vi "IniDataRd TDC.vi"(8 "error in":errorcluster, 10 "MODBUS section":string="Modbus", 11 "INI file path":path=path "C:/Users/User/Desktop/YDX701_TDC/iniData/TDC_IniData.ini") -> (0 "error out":errorcluster, 2 "MODBUS Para":T1={"COMPort"="COM4", "Slave Address"=1, " Baud"=9600, "Timeout"=100})   [LabVIEW 2019]
uses:
  <vilib>/Utility/config.llb/Read Key (U32).vi
  <vilib>/Utility/config.llb/Read Key (String).vi
  <vilib>/Utility/config.llb/NI_LVConfig.lvlib
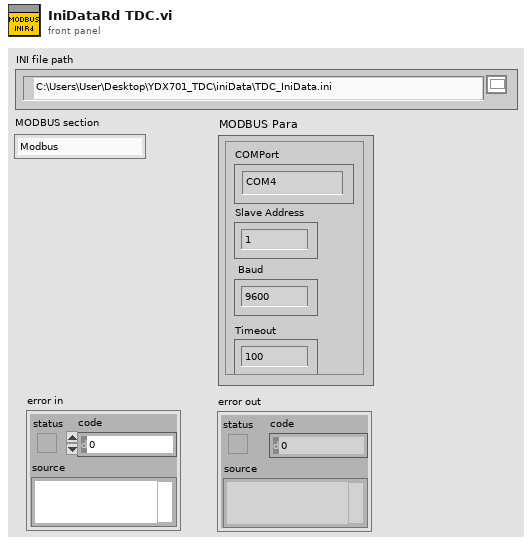
[diagram p1: front panel]
types:
  T1 = cluster{"COMPort":string, "Slave Address":u32, " Baud":u32, "Timeout":u32}
  T2 = typedef "NI_LVConfig.lvlib/Config Data RefNum.ctl" = refnum<k1>
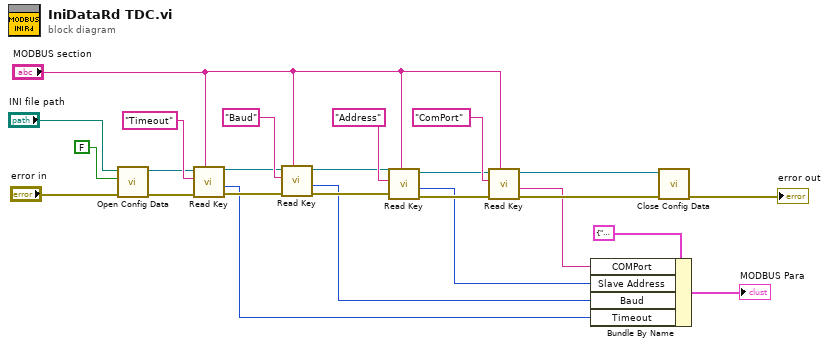
[diagram p0: block diagram]
diagram:
  n1 = call <vilib>:"Open Config Data.vi"("error in (no error)"="error in", "create file if necessary (T)"=FALSE ("create file if necessary? (T)"), "configuration file path"="INI file path") -> ("error out"=w23:errorcluster, "refnum"=w21:T2)  [unwired: 6 in, 1 out]
  n2 = call-poly <vilib>:"Read Key.vi"("section"="MODBUS section", "error in (no error)"=w23, "key"="Timeout", "refnum"=w21) -> ("error out"=w7:errorcluster, "value"=w1:u32, "refnum out"=w9:T2)  [unwired: 1 in, 4 out]
  n3 = call-poly <vilib>:"Read Key.vi"("section"="MODBUS section", "error in (no error)"=w7, "key"="Baud", "refnum"=w9) -> ("error out"=w6:errorcluster, "value"=w2:u32, "refnum out"=w8:T2)  [unwired: 1 in, 4 out]
  n4 = call-poly <vilib>:"Read Key.vi"("section"="MODBUS section", "error in (no error)"=w6, "key"="Address", "refnum"=w8) -> ("error out"=w12:errorcluster, "value"=w3:u32, "refnum out"=w13:T2)  [unwired: 1 in, 4 out]
  n5 = call-poly <vilib>:"Read Key.vi"("section"="MODBUS section", "error in (no error)"=w12, "key"="ComPort", "refnum"=w13) -> ("error out"=w18:errorcluster, "value"=w10:string, "refnum out"=w19:T2)  [unwired: 2 in, 3 out]
  n6 = Bundle By Name(cluster=T1 {"COMPort"="COM4", "Slave Address"=1, " Baud"=9600, "Timeout"=100} ("MODBUS Para 2"), "COMPort"=w10, "Slave Address"=w3, "Baud"=w2, "Timeout"=w1) -> (→"MODBUS Para":T1)
  n7 = call <vilib>:"Close Config Data.vi"("error in (no error)"=w18, "refnum"=w19) -> ("error out"=→"error out":errorcluster)  [unwired: 1 in, 8 out]
